vi "Read Path To Filter.vi"(9 "VI Name":T1) -> (1 "vi path":path)   [LabVIEW 2019]
doc: "A VI to generate the path to the dynamically loaded filter subVIs used in one lesson of this tutorial."
uses:
  Noise Enum.ctl
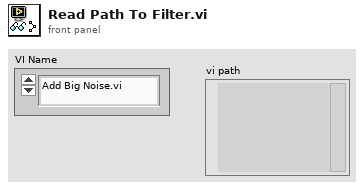
[diagram p1: front panel]
types:
  T1 = typedef "Noise Enum.ctl" = enum16{"Add Big Noise.vi", "Add Small Noise.vi"}
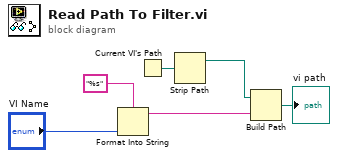
[diagram p0: block diagram]
diagram:
  n1 = Format Into String(format string="%s", "VI Name") -> (resulting string=w3:string)  [unwired: 2 in, 1 out]
  n2 = Current VI's Path() -> (path=w4:path)
  n3 = Strip Path(path=w4) -> (stripped path=w1:path)  [unwired: 1 out]
  n4 = Build Path(base path=w1, name or relative path=w3) -> (appended path=→"vi path":path)
